vi "OP400ZP_prep bdd ocvacir.vi"(8 "tabin":string[](array[string]), 11 "DataStr":cluster{"Rstr":string, "Vstr":string}) -> (0 "tabout":string[](array[string]))   [LabVIEW 2020]
uses:
  CtrldeTest/selectdata.ctl
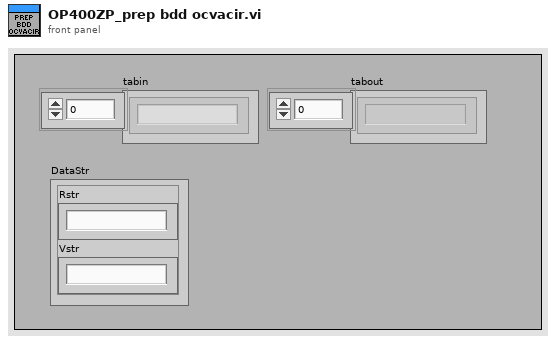
[diagram p1: front panel]
types:
  T1 = typedef "selectdata.ctl" = u16
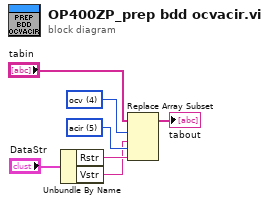
[diagram p0: block diagram]
diagram:
  w7 = T1 5 items=["id", "date", "type", "sn", "ocv", "acir", "insuP", "insuN", "TC01", "TC02", "TC11", "TC12", "TC21", "TC22", "VC01", "VC02", "VC03", "VC04", "VC11", "VC12", "VC13", "VC14", "VC21", "VC22", "VC23", "VC24", "DCIRN", "DCIRP", "inifilevers", "softvers", "imagevers", "pass", "operateur", "tpstest"] ("Menu déroulant")
  w1 = T1 4 items=["id", "date", "type", "sn", "ocv", "acir", "insuP", "insuN", "TC01", "TC02", "TC11", "TC12", "TC21", "TC22", "VC01", "VC02", "VC03", "VC04", "VC11", "VC12", "VC13", "VC14", "VC21", "VC22", "VC23", "VC24", "DCIRN", "DCIRP", "inifilevers", "softvers", "imagevers", "pass", "operateur", "tpstest"] ("Menu déroulant")
  n1 = Unbundle By Name("DataStr") -> ("Rstr"=w6:string, "Vstr"=w4:string)
  n2 = Replace Array Subset(array="tabin", new element #1=w4, index #1=w1, new element #2=w6, index #2=w7) -> (→"tabout":string[])
